vi "Write and Read Multiple Registers.vi"(4 "read count":u16, 6 "read starting address":u16, 8 "error in (no error)":errorcluster, 9 "write values":u16[](array[numeric]), 10 "write starting address":u16, 11 "device data model in":refnum<class "ICPCON ET Data Model.lvclass">) -> (0 "error out":errorcluster, 1 "read values":u16[](array[numeric]), 3 "device data model out":refnum<class "ICPCON ET Data Model.lvclass">)   [LabVIEW 2021, in "ICPCON ET Data Model.lvclass"]
doc: "Writes and reads the values of multiple register values in series. The <b>write values</b> are inserted starting at <b>write starting address</b> and the returned <b>read values</b> consists of <b>read count</b> holding registers starting at <b>read starting address</b>."
uses:
  ICPCON ET Data Model.lvclass
  ICPCON ET Data Model.lvclass/ICPCON ET Data Model.ctl
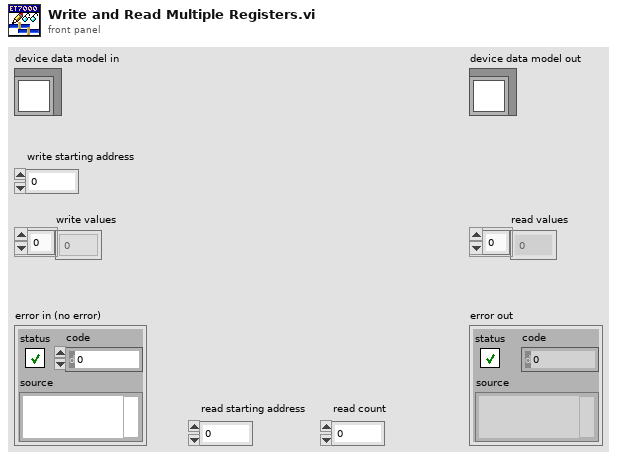
[diagram p1: front panel]
types:
  T1 = typedef "SubVIs.lvlib/ICPCON ET Data Model.lvclass/Data Model.ctl" = cluster{"UTC":u64, "DI":bool[], "DO":bool[], "IR":u16[], "HR":u16[], "ES":u8}
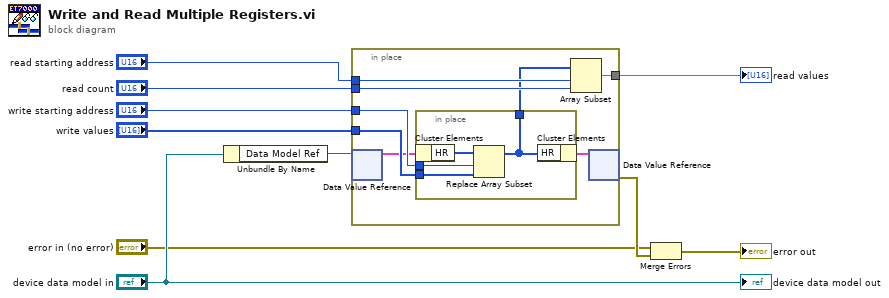
[diagram p0: block diagram]
diagram:
  n1 = Unbundle By Name("device data model in") -> ("Data Model Ref"=w3:refnum<data-value>)
  n2 = in-place {
    in-place-border: "write values" -> [w18]
    in-place-border: "write starting address" -> [w17]
    in-place-border: [w16] -> w7
    in-place-border: "read count" -> [w14]
    in-place-border: "read starting address" -> [w15]
    n3 = in-place-dvr #1(w3) -> (w13:T1)  [unwired: 1 out]
    n4 = in-place {
      in-place-border: w18 -> [w22]
      in-place-border: w17 -> [w21]
      in-place-border: [w19] -> w11
      n5 = in-place-cluster #2(w13) -> ("HR"=w20:u16[])
      n6 = Replace Array Subset(array=w20, new element=w22, index=w21) -> (w19:u16[])
      n7 = in-place-cluster #2("HR"=w19) -> (w12:T1)
    }
    n8 = Array Subset(array=w11, index=w15, length=w14) -> (w16:u16[])
    n9 = in-place-dvr #1(w12) -> (w2:errorcluster)  [unwired: 1 out]
  }
  "read values" <- w7
  n10 = Merge Errors("error in (no error)", w2) -> (→"error out":errorcluster)
  "device data model out" <- "device data model in"
